vi "Add_to_sequence_SubVI_Directly.vi"(1 "Delay [us]":dbl, 2 "Pulse length [us]":dbl, 3 "Channel number":i32, 4 "Array sequence in":cluster{"Timing 0":dbl[]}[](array[cluster])) -> (0 "Array sequence out":cluster{"Timing 0":dbl[]}[](array[cluster]))   [LabVIEW 2021]
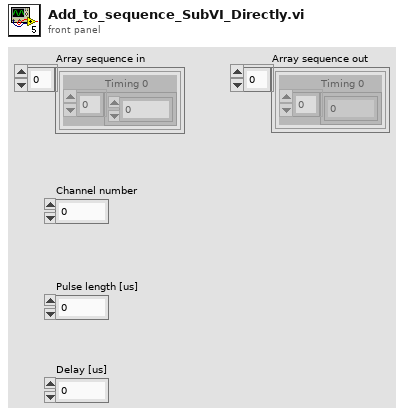
[diagram p1: front panel]
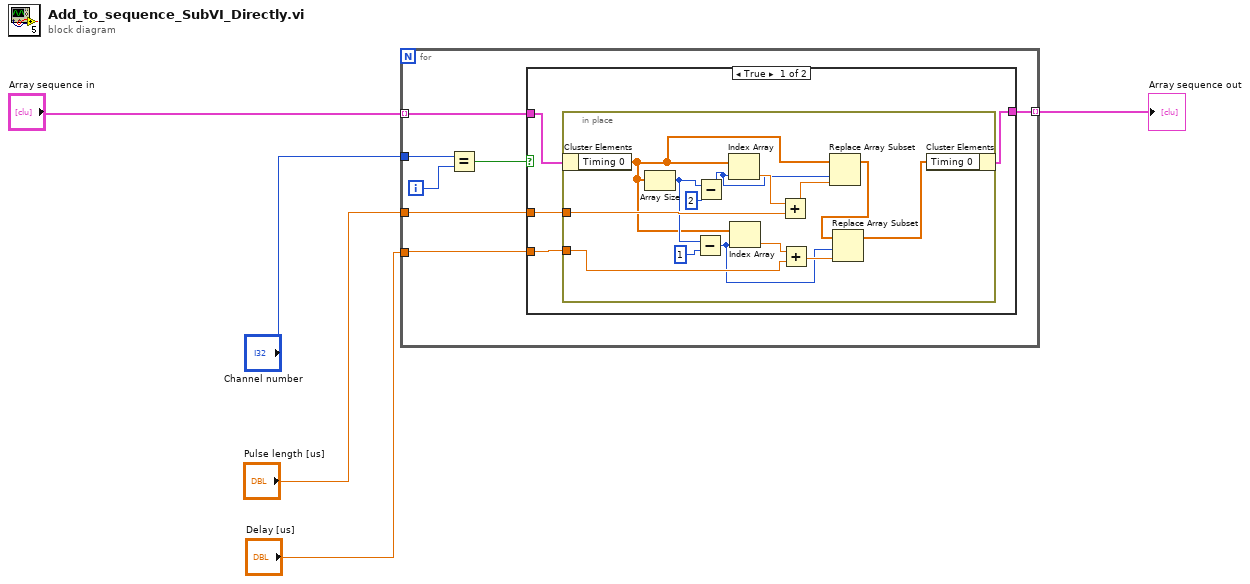
[diagram p0: block diagram]
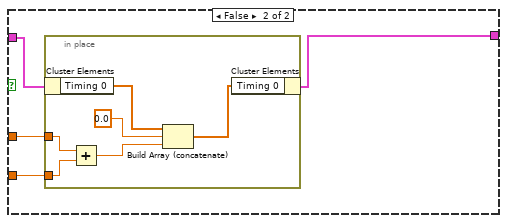
[diagram p2: hidden frame]
diagram:
  n1 = for {
    tunnel: "Array sequence in" -> [w9] mode=indexing
    tunnel: "Channel number" -> [w12]
    tunnel: "Pulse length [us]" -> [w8]
    tunnel: [w7] -> w5 mode=indexing
    tunnel: "Delay [us]" -> [w6]
    i -> [w11]
    n2 = Equal?(x=w12, y=w11) -> (x = y?=w10:bool)
    n3 = case shown="True" w10 {
      tunnel: w9 -> [w16 w34]
      tunnel: w8 -> [w15 w33]
      tunnel: [w14 w32] -> w7
      tunnel: w6 -> [w13 w31]
      frame True {
        n4 = in-place {
          in-place-border: w15 -> [w29]
          in-place-border: w13 -> [w22]
          n5 = in-place-cluster #1(w16) -> ("Timing 0"=w21:dbl[])
          n6 = Array Size(array=w21) -> (size(s)=w25:i32)
          n7 = Subtract(x=w25, y=1) -> (x-y=w19:i32)
          n8 = Subtract(x=w25, y=2) -> (x-y=w27:i32)
          n9 = Index Array(array=w21, index=w27) -> (element=w30:dbl)
          n10 = Index Array(array=w21, index=w19) -> (element=w23:dbl)
          n11 = Add(x=w30, y=w29) -> (x+y=w28:dbl)
          n12 = Add(x=w23, y=w22) -> (x+y=w20:dbl)
          n13 = Replace Array Subset(array=w21, new element=w28, index=w27) -> (w18:dbl[])
          n14 = Replace Array Subset(array=w18, new element=w20, index=w19) -> (w17:dbl[])
          n15 = in-place-cluster #1("Timing 0"=w17) -> (w14:cluster{"Timing 0":dbl[]})
        }
      }
      frame False {
        n16 = in-place {
          in-place-border: w33 -> [w37]
          in-place-border: w31 -> [w36]
          n17 = in-place-cluster #2(w34) -> ("Timing 0"=w40:dbl[])
          n18 = Add(x=w37, y=w36) -> (x+y=w35:dbl)
          n19 = Build Array (concatenate)(w40, 0.0 ("element"), w35) -> (w39:dbl[])
          n20 = in-place-cluster #2("Timing 0"=w39) -> (w32:cluster{"Timing 0":dbl[]})
        }
      }
    }
  }
  "Array sequence out" <- w5
